vi "labview_python.vi"(9 "current state":i32[][](array[numeric]), 11 "input":i32[][](array[numeric])) -> (0 "return value 4":i32[][](array[numeric]))   [LabVIEW 2021]
panel:
  out "py_ver":string="3.8"
  out "return value 3":string
  out "Array":string[][](array[string])
  out "error out":errorcluster
  in  "error in (no error)":errorcluster
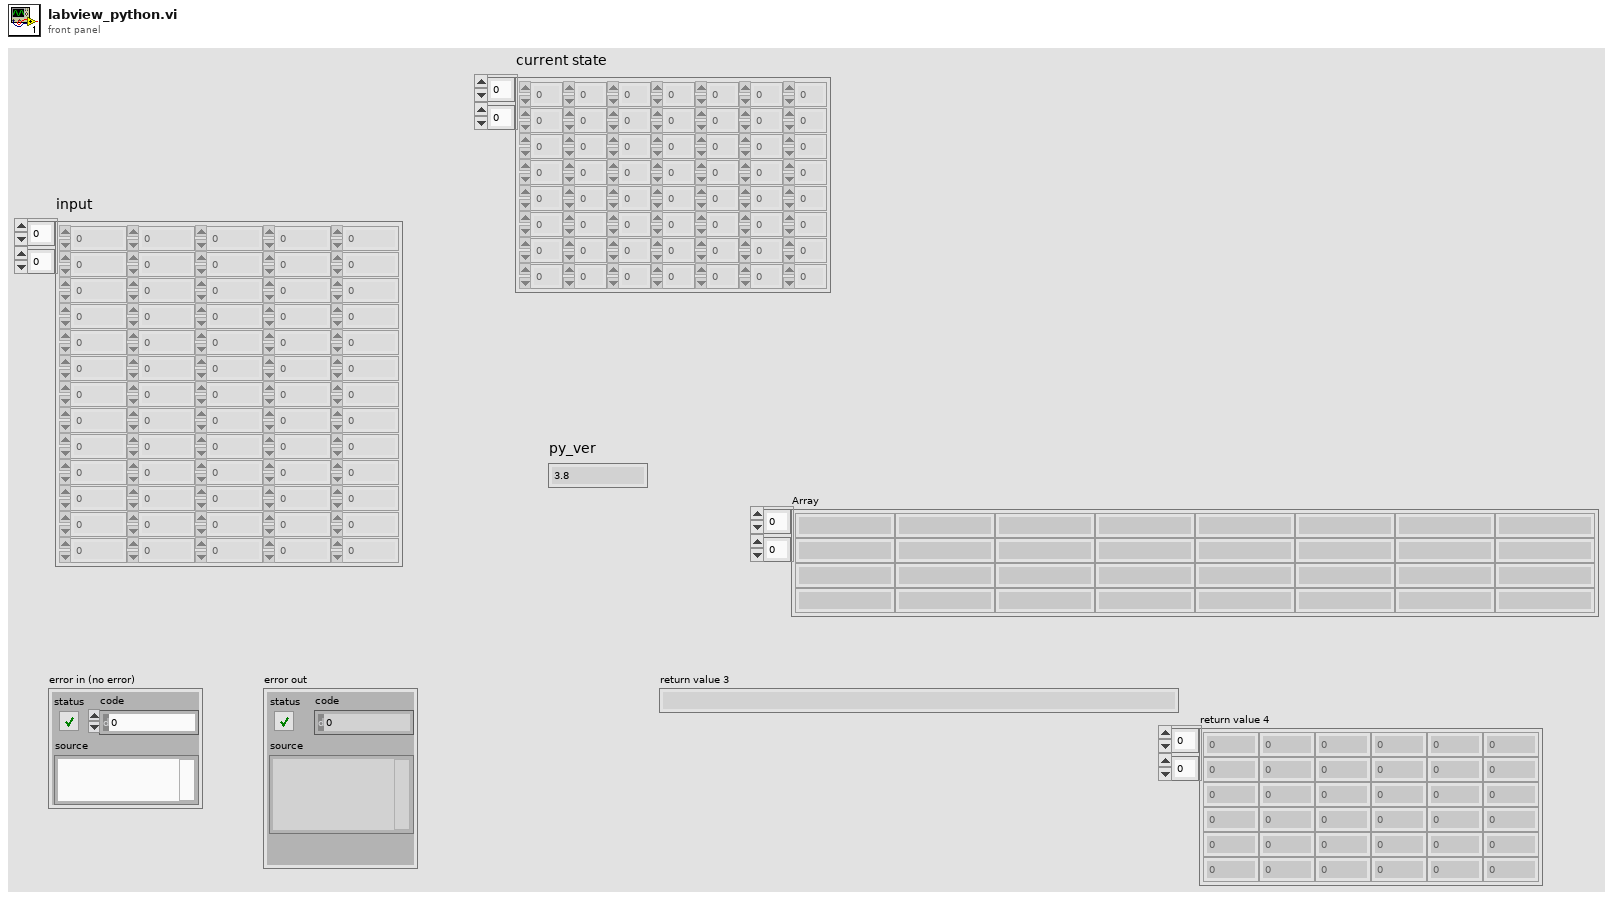
[diagram p1: front panel]
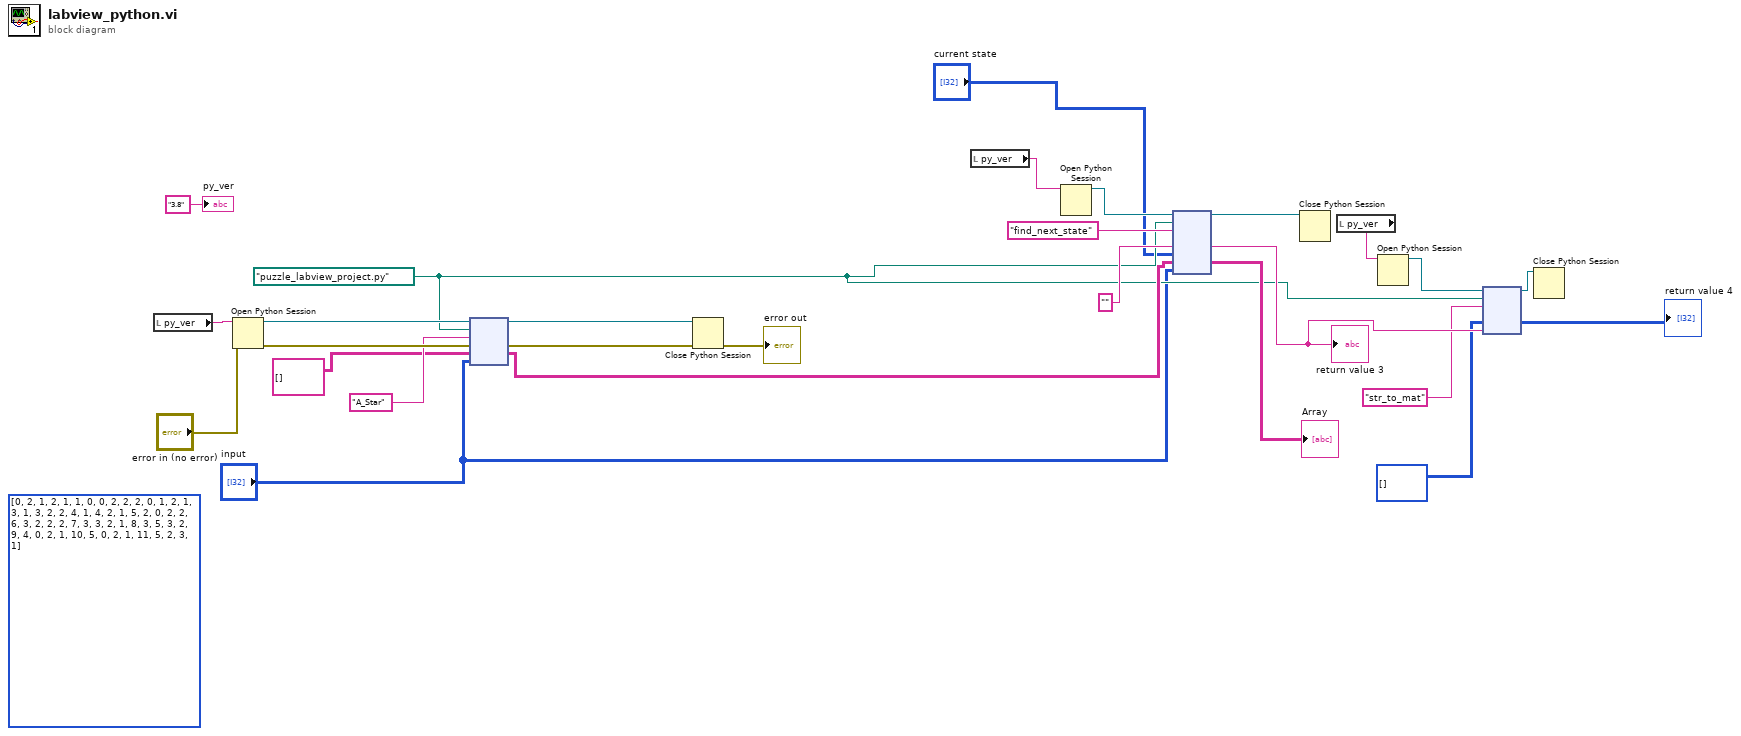
[diagram p0: block diagram]
diagram:
  (unwired) i32[][] [[0, 2, 1, 2, 1], [1, 0, 0, 2, 2], [2, 0, 1, 2, 1], [3, 1, 3, 2, 2], [4, 1, 4, 2, 1], [5, 2, 0, 2, 2], [6, 3, 2, 2, 2], [7, 3, 3, 2, 1], [8, 3, 5, 3, 2], [9, 4, 0, 2, 1], [10, 5, 0, 2, 1], [11, 5, 2, 3, 1]]
  w10 = path "puzzle_labview_project.py" ("module path")
  n1 = local read "py_ver"() -> (w5:string)
  n2 = Open Python Session(python version=w5, 3:"error in (no error)") -> (session out=w20:refnum<k35>, error out=w26:errorcluster)  [unwired: 1 in]
  n3 = node(w20, w10, "A_Star" ("function name"), w26, string[][] [], "input") -> (w21:refnum<k35>, w24:errorcluster, w16:string[][])  [unwired: 1 in, 2 out]
  n4 = Close Python Session(session in=w21, error in=w24) -> (11:→"error out":errorcluster)
  n5 = local read "py_ver"() -> (w4:string)
  n6 = Open Python Session(python version=w4) -> (session out=w19:refnum<k35>)  [unwired: 2 in, 1 out]
  n7 = node(w19, w10, "find_next_state" ("function name"), "", "current state", w16, "input") -> (w18:refnum<k35>, w13:string, →"Array":string[][])  [unwired: 3 in, 3 out]
  "return value 3" <- w13
  n8 = Close Python Session(session in=w18) -> ()  [unwired: 1 in, 1 out]
  n9 = local read "py_ver"() -> (w3:string)
  n10 = Open Python Session(python version=w3) -> (session out=w12:refnum<k35>)  [unwired: 2 in, 1 out]
  n11 = node(w12, w10, "str_to_mat" ("function name"), i32[][] [], w13) -> (w11:refnum<k35>, →"return value 4":i32[][])  [unwired: 2 in, 3 out]
  n12 = Close Python Session(session in=w11) -> ()  [unwired: 1 in, 1 out]
  "py_ver" <- "3.8"
